vi "Create Listener.vi"(8 "error in (no error)":errorcluster, 9 "timeout ms (5000)":i32=5000, 10 "Port":u16, 11 "dotNET Listener in":refnum<class "dotNET Listener.lvclass">) -> (0 "error out":errorcluster, 3 "dotNET Listener out":refnum<class "dotNET Listener.lvclass">)   [LabVIEW 2013, in "dotNET SSL Socket.lvlib" / "dotNET Listener.lvclass"]
uses:
  dotNET Listener.lvclass
  dotNET Listener.lvclass/dotNET Listener.ctl
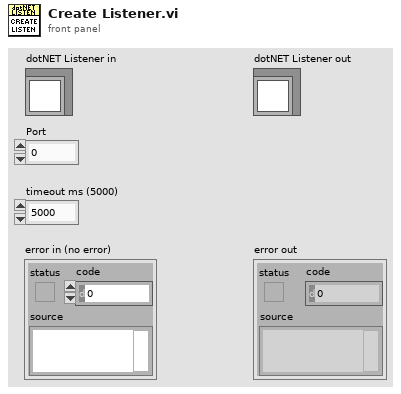
[diagram p1: front panel]
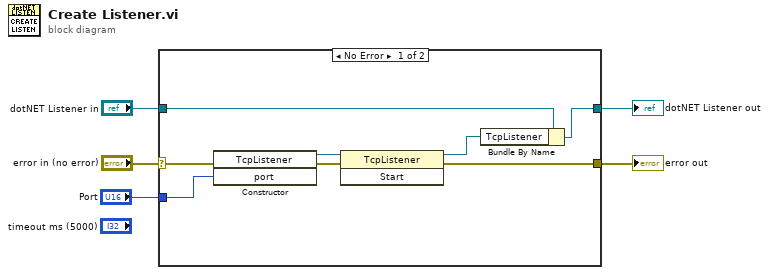
[diagram p0: block diagram]
diagram:
  n1 = case shown="No Error" "error in (no error)" {
    selector: "error in (no error)" -> [w11 w15]
    tunnel: [w10 w15] -> w4
    tunnel: [w7 w14] -> w3
    tunnel: "dotNET Listener in" -> [w8 w14]
    tunnel: "Port" -> [w9 _]
    frame No Error {
      n2 = constructor class="TcpListener"(error in=w11, "port"=w9) -> (reference out=w13:refnum<k24>, error out=w12:errorcluster)  [unwired: 2 in, 2 out]
      n3 = invoke class="TcpListener" method="Start"(reference=w13, error in=w12) -> (reference out=w6:refnum<k24>, error out=w10:errorcluster)  [unwired: 1 in, 1 out]
      n4 = Bundle By Name(cluster=w8, "TcpListener"=w6) -> (w7:refnum<class "dotNET Listener.lvclass">)
    }
    frame Error {
    }
  }
  "error out" <- w4
  "dotNET Listener out" <- w3
